vi "Ad_.vi"(11 "X":dbl) -> (3 "X'":dbl)   [LabVIEW 2017]
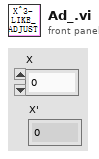
[diagram p1: front panel]
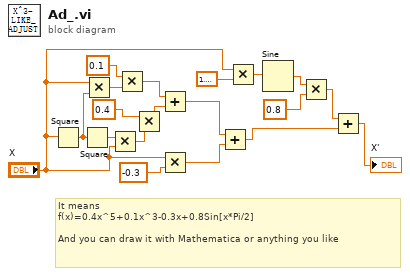
[diagram p0: block diagram]
diagram:
  # "It means\nf(x)=0.4x^5+0.1x^3-0.3x+0.8Sin[x*Pi/2]\n\nAnd you can draw it with Mathematica or anything you like"
  n1 = Square(x="X") -> (x^2=w16:dbl)
  n2 = Square(x=w16) -> (x^2=w19:dbl)
  n3 = Multiply(x="X", y=w16) -> (x*y=w15:dbl)
  n4 = Multiply(x=w19, y="X") -> (x*y=w18:dbl)
  n5 = Multiply(x=0.1, y=w15) -> (x*y=w13:dbl)
  n6 = Multiply(x=0.4, y=w18) -> (x*y=w12:dbl)
  n7 = Add(x=w13, y=w12) -> (x+y=w11:dbl)
  n8 = Multiply(x="X", y=-0.3) -> (x*y=w10:dbl)
  n9 = Add(x=w11, y=w10) -> (x+y=w4:dbl)
  n10 = Multiply(x="X", y=1.5707963267948966) -> (x*y=w7:dbl)
  n11 = Sine(x=w7) -> (sin(x)=w6:dbl)
  n12 = Multiply(x=w6, y=0.8) -> (x*y=w3:dbl)
  n13 = Add(x=w3, y=w4) -> (x+y=→"X'":dbl)
